vi "SiosIfmSetFilter.vi"(1 "AVG2":u8, 2 "AVG1":u8, 3 "FilterFlag":u32, 4 "DeviceNumber":i32) -> (0 "success":i32)   [LabVIEW 2009]
uses:
  siosifm.dll
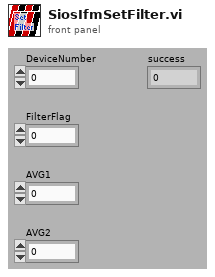
[diagram p1: front panel]
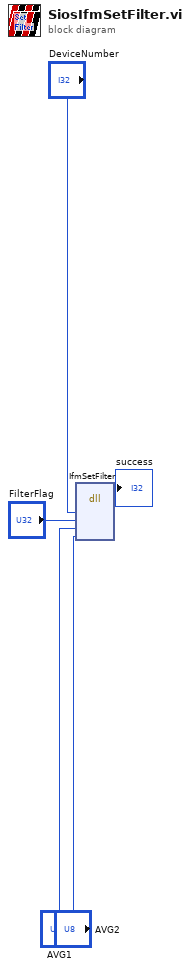
[diagram p0: block diagram]
diagram:
  n1 = dll-call lib="D:/Support/Labview/RE-10/SIOS_IfmDLL/siosifm.dll" fn="IfmSetFilter"("deviceNumber"="DeviceNumber", "filterFlags"="FilterFlag", "avg1"="AVG1", "avg2"="AVG2") -> (→"success":i32)  [unwired: 7 in, 2 out]
